vi "depth read 2016.vi"(0 "Debug":bool, 1 "Initialize Debug":bool, 2 "Read String Pot":bool=TRUE, 3 "Increment Button":bool, 4 "Descriptions":string[](array[string]), 5 "error in (no error)":errorcluster, 6 "String Pot \nSlope":dbl=1.7339999675750732 format="%.2f", 10 "Array in":refnum<k24>[](array[refnum]), 11 "Sensor Cluster In":T1) -> (12 "Array out":refnum<k24>[](array[refnum]), 13 "Sensor Cluster 2":T1, 14 "Depth":dbl format="%.2f", 19 "error out":errorcluster)   [LabVIEW 2016]
uses:
  Waterloo DAQ/controls/MCC DAQ Readings.ctl
  C:/Program Files (x86)/National Instruments/LabVIEW 2016/vi.lib/ULx/ULx_LV.dll
  KPRO_lv2015/ad interface/Global_SIM_switch.vi
  KPRO_lv2015/Kpro Globals.vi
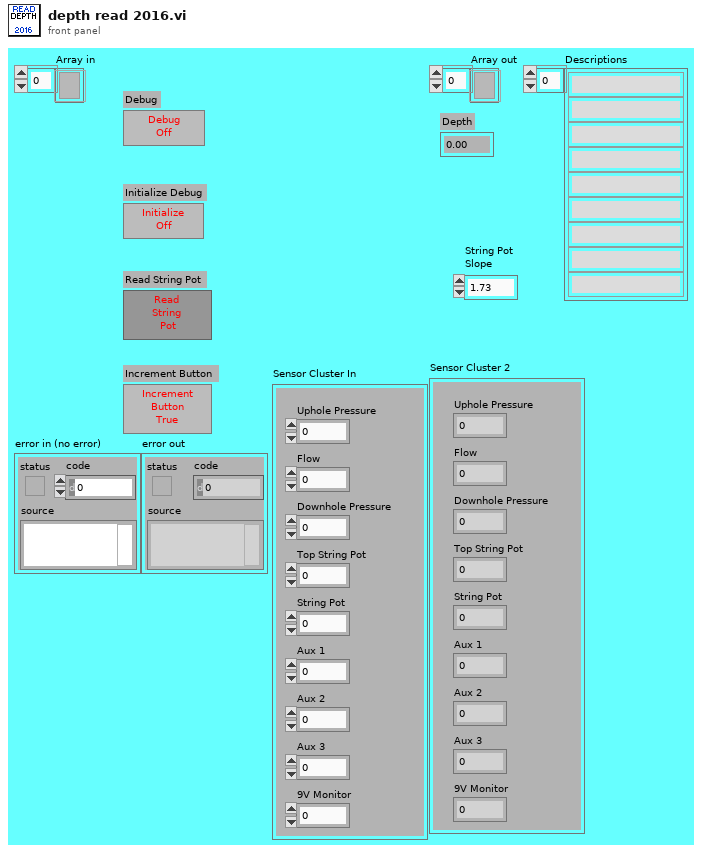
[diagram p1: front panel]
types:
  T1 = typedef "MCC DAQ Readings.ctl" = cluster{"Uphole Pressure":dbl, "Flow":dbl, "Downhole Pressure":dbl, "Top String Pot":dbl, "String Pot":dbl, "Aux 1":dbl, "Aux 2":dbl, "Aux 3":dbl, "9V Monitor":dbl}
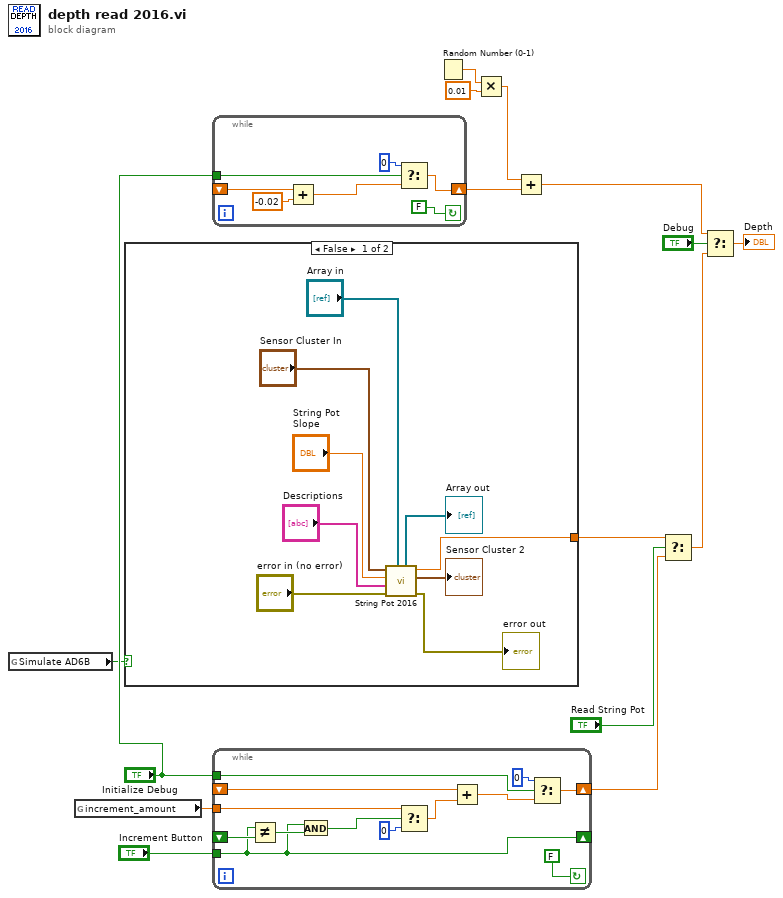
[diagram p0: block diagram]
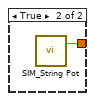
[diagram p2: hidden frame]
diagram:
  n1 = global read "Global_SIM_switch.vi" "Simulate AD6B"() -> (w2:bool)
  n2 = global read "Kpro Globals.vi" "increment_amount"() -> (w1:dbl)
  n3 = case shown="False" w2 {
    tunnel: [w24 w25] -> w3
    frame False {
      n4 = call "String Pot 2016.vi"("Array in"="Array in", "error in (no error)"="error in (no error)", "Descriptions"="Descriptions", "String Pot \nSlope"="String Pot \nSlope", "Sensor Cluster"="Sensor Cluster In") -> ("error out"=→"error out":errorcluster, "Sensor Cluster 2"=→"Sensor Cluster 2":T1, "Distance (in)"=w24:dbl, "Array out"=→"Array out":refnum<k24>[])  [unwired: 3 in]
    }
    frame True {
      n5 = call "SIM_String Pot.vi"() -> ("Distance (in)"=w25:dbl)  [unwired: 3 in]
    }
  }
  n6 = while {
    tunnel: "Initialize Debug" -> [w31]
    shift-left: _ -> [w29]
    shift-right: [w30] -> w13
    stop <- FALSE continue-if-true
    n7 = Add(x=w29, y=-0.02) -> (x+y=w27:dbl)
    n8 = Select(t=0, s=w31, f=w27) -> (s? t:f=w30:dbl)
  }
  n9 = while {
    tunnel: w1 -> [w33]
    tunnel: "Increment Button" -> [w35]
    shift-left: _ -> [w40]
    shift-right: [w35] -> _
    tunnel: "Initialize Debug" -> [w41]
    shift-left: _ -> [w43]
    shift-right: [w44] -> w4
    stop <- FALSE continue-if-true
    n10 = Not Equal?(x=w35, y=w40) -> (x != y?=w38:bool)
    n11 = And(x=w35, y=w38) -> (x .and. y?=w36:bool)
    n12 = Select(t=w33, s=w36, f=0) -> (s? t:f=w39:dbl)
    n13 = Add(x=w43, y=w39) -> (x+y=w42:dbl)
    n14 = Select(t=0, s=w41, f=w42) -> (s? t:f=w44:dbl)
  }
  n15 = Random Number (0-1)() -> (number: 0 to 1=w15:dbl)
  n16 = Multiply(x=w15, y=0.01) -> (x*y=w12:dbl)
  n17 = Add(x=w12, y=w13) -> (x+y=w9:dbl)
  n18 = Select(t=w3, s="Read String Pot", f=w4) -> (s? t:f=w8:dbl)
  n19 = Select(t=w9, s="Debug", f=w8) -> (s? t:f=→"Depth":dbl)
